vi "CreateDiagrams.vi"(6 "error in":errorcluster, 9 "Structure in":refnum<class "Structure.lvclass">) -> (0 "error out":errorcluster, 3 "Structure out":refnum<class "Structure.lvclass">, 4 "create_diagrams":string)   [LabVIEW 2014, in "Raspberry Pi Compatible Compiler for LabVIEW.lvlib" / "Structure.lvclass"]
uses:
  Structure.lvclass
  Python/Parsing/ClassTypeTD.ctl
  Python/Parsing/ListTypesTD.ctl
  Structure.lvclass/Structure.ctl
  Diagram/Diagram.lvclass
  Python/Parsing/Python Functions.lvlib
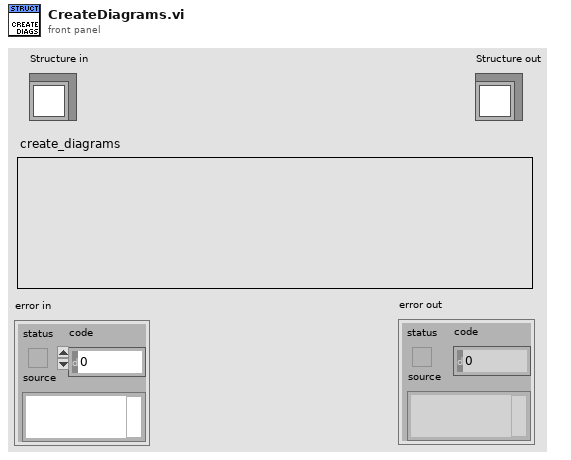
[diagram p1: front panel]
types:
  T1 = typedef "Raspberry Pi Compatible Compiler for LabVIEW.lvlib/Python Functions.lvlib/ListTypesTD.ctl" = enum16{"list", "tuple", "parameter list", "output list", "return values"}
  T2 = typedef "Raspberry Pi Compatible Compiler for LabVIEW.lvlib/Python Functions.lvlib/ClassTypeTD.ctl" = enum16{"class", "function"}
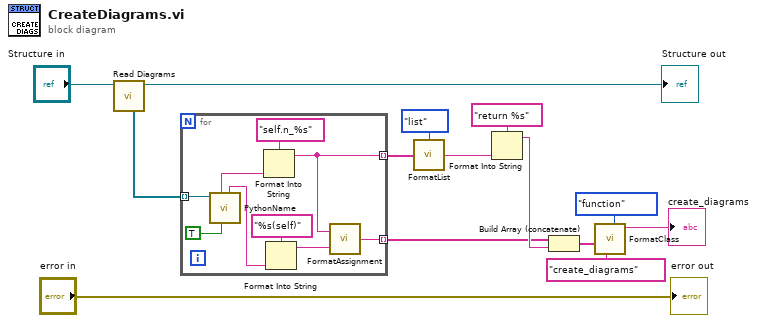
[diagram p0: block diagram]
diagram:
  n1 = call "Read Diagrams.vi"("Structure in"="Structure in") -> ("Structure out"=→"Structure out":refnum<class "Structure.lvclass">, "Diagrams"=w13:refnum<class "Diagram.lvclass">[])  [unwired: 7 in]
  n2 = for {
    tunnel: w13 -> [w23] mode=indexing
    tunnel: [w17] -> w8 mode=indexing
    tunnel: [w15] -> w3 mode=indexing
    n3 = call-dynamic "PythonName.vi"("add self"=TRUE, "Diagram in"=w23) -> ("name"=w18:string, "UID"=w20:string)  [unwired: 6 in, 2 out]
    n4 = Format Into String(format string="self.n_%s", w20) -> (resulting string=w17:string)  [unwired: 2 in, 1 out]
    n5 = Format Into String(format string="%s(self)", w18) -> (resulting string=w16:string)  [unwired: 2 in, 1 out]
    n6 = call "FormatAssignment.vi"("value"=w16, "name"=w17) -> ("python assignment"=w15:string)
  }
  n7 = call "FormatList.vi"("values"=w8, "type"=ListTypesTD."list") -> ("python object"=w6:string)
  n8 = Format Into String(format string="return %s", w6) -> (resulting string=w4:string)  [unwired: 2 in, 1 out]
  n9 = Build Array (concatenate)(w3, w4) -> (w1:string[])
  n10 = call "FormatClass.vi"("type"=ClassTypeTD."function", "name"="create_diagrams", "body"=w1) -> ("python"=→"create_diagrams":string)  [unwired: 8 in]
  "error out" <- "error in"
